vi "Build Name and Value arrays from Variant.vi"(7 "Format String (%#_13g)":string="%.3f", 8 "Error":errorcluster, 11 "Anything":variant) -> (0 "Error Out":errorcluster, 2 "Value Array Out":string[](array[string]), 3 "Name Array Out":string[](array[string]), 5 "Default Section Name Out":string)   [LabVIEW 2020]
uses:
  <vilib>/Utility/Data Type/NI_Data Type.lvlib
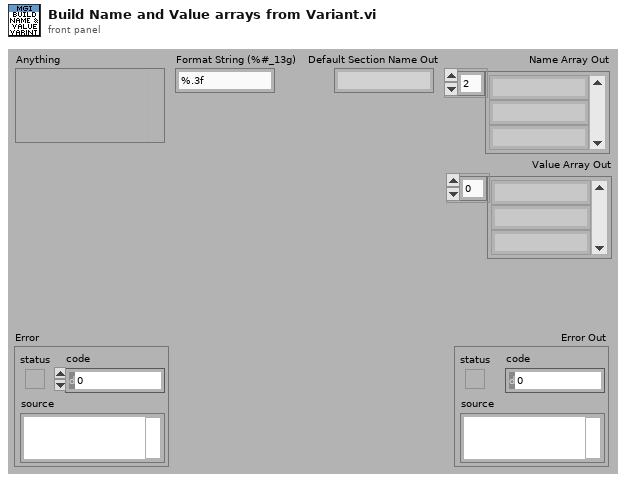
[diagram p1: front panel]
types:
  T1 = typedef "NI_Data Type.lvlib/Data Type.ctl" = enum8{"Invalid Type", "Void", "I8", "I16", "I32", "I64", "U8", "U16", "U32", "U64", "Single Float", "Double Float", "Extended Float", "Single Complex", "Double Complex", "Extended Complex", "Enum U8", "Enum U16", "Enum U32", "Enum U64", "Single Float With Unit", "Double Float With Unit", "Extended Float With Unit", "Single Complex with Unit", "Double Complex with Unit", "Extended Complex with Unit", "Boolean", "String", "Path", "Picture", "Tag", "Array", "Cluster", "Variant", "LV Variant", "Waveform", "Timestamp", "Digital Waveform", "Digital Data", "ExpressData", "Refnum", "External Data", "VI", "Poly VI", "LabVIEW Class Instance", "Fixed Point", "Set Collection", "Map Collection"}
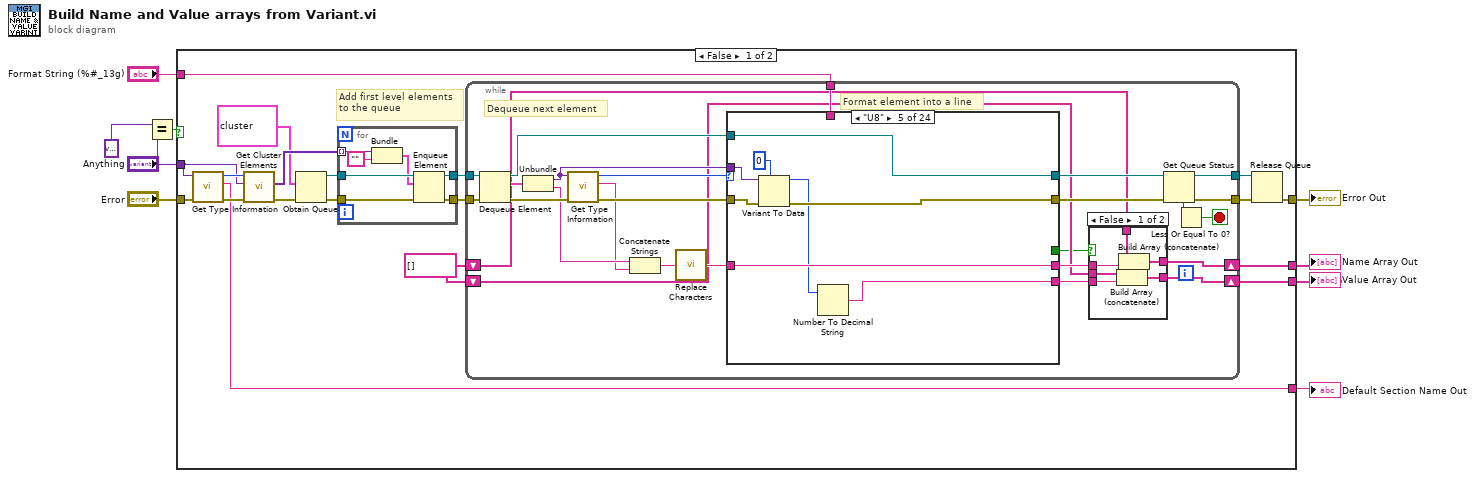
[diagram p0: block diagram]
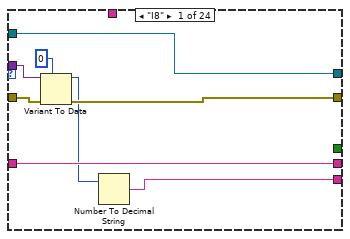
[diagram p3: hidden frame]
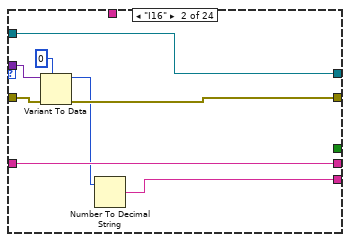
[diagram p4: hidden frame]
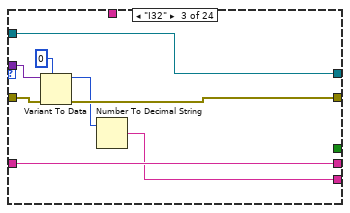
[diagram p5: hidden frame]
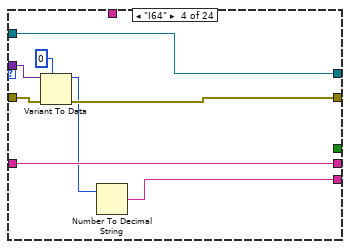
[diagram p6: hidden frame]
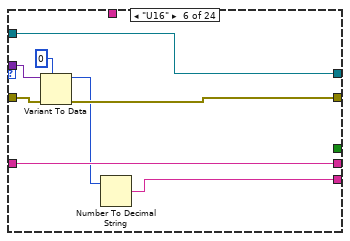
[diagram p7: hidden frame]
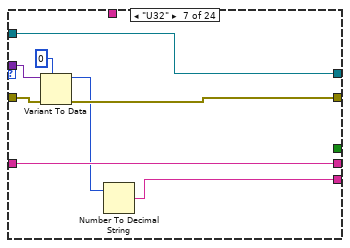
[diagram p8: hidden frame]
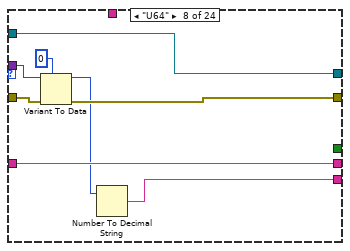
[diagram p9: hidden frame]
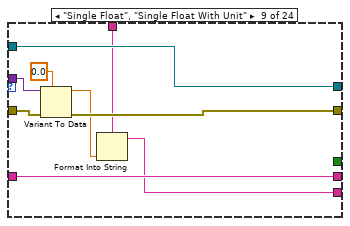
[diagram p10: hidden frame]
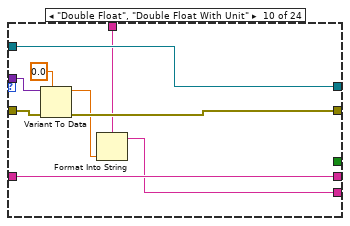
[diagram p11: hidden frame]
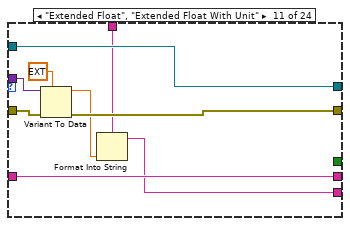
[diagram p12: hidden frame]
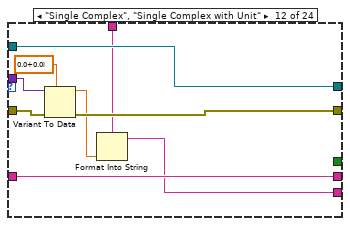
[diagram p13: hidden frame]
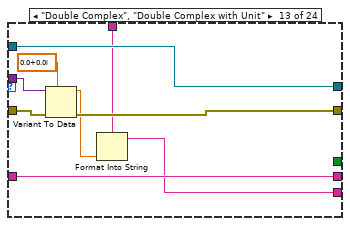
[diagram p14: hidden frame]
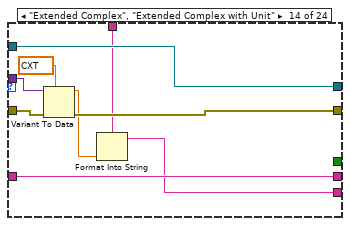
[diagram p15: hidden frame]
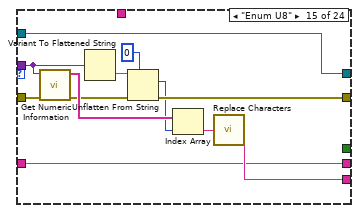
[diagram p16: hidden frame]
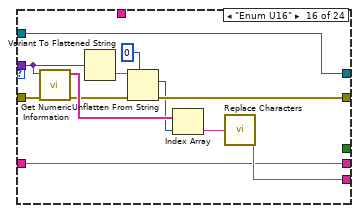
[diagram p17: hidden frame]
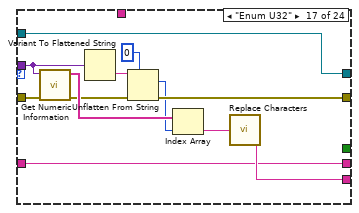
[diagram p18: hidden frame]
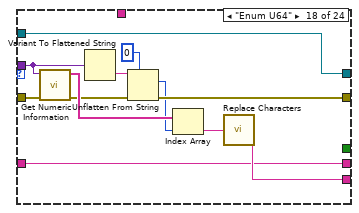
[diagram p19: hidden frame]
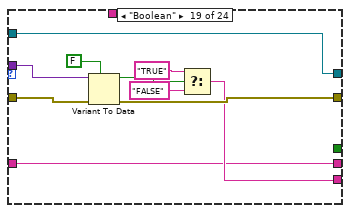
[diagram p20: hidden frame]
diagram:
  n1 = Equal?(x=variant ("Anything"), y="Anything") -> (x = y?=w1:bool)
  n2 = case shown="False" w1 {
    tunnel: [w28 _] -> w9
    tunnel: [w27 _] -> w8
    tunnel: "Error" -> [w26 w301]
    tunnel: "Format String (%#_13g)" -> [w25 _]
    tunnel: [w23 w301] -> w5
    tunnel: [w12 _] -> w4
    tunnel: "Anything" -> [w10 _]
    frame False {
      w11 = string[] []
      # "Add first level elements\nto the queue"
      n3 = call <vilib>:"Get Type Information.vi"("error in (no error)"=w26, "variant"=w10) -> ("error out"=w20:errorcluster, "name"=w12:string, "type"=w24:T1)  [unwired: 5 in, 2 out]
      n4 = call "Get Cluster Elements.vi"("Error In"=w20, "Cluster"=w10, "Type Enum (Cluster)"=w24) -> ("Error Out"=w22:errorcluster, "Cluster Elements"=w21:variant[])  [unwired: 7 in]
      n5 = Obtain Queue(element data type=cluster{"Variant":variant, "Name":string} {"Variant"=variant, "Name"=""}, error in (no error)=w22) -> (queue out=w13:refnum<queue>, error out=w14:errorcluster)  [unwired: 3 in, 1 out]
      n6 = for {
        tunnel: w13 -> [w35]
        tunnel: w14 -> [w34]
        tunnel: [w33] -> w15
        tunnel: [w32] -> w16
        tunnel: w21 -> [w30] mode=indexing
        n7 = Bundle("Variant"=w30, "") -> (w31:cluster{"Variant":variant, string})  [unwired: 1 in]
        n8 = Enqueue Element(queue=w35, element=w31, error in (no error)=w34) -> (queue out=w32:refnum<queue>, error out=w33:errorcluster)  [unwired: 1 in, 1 out]
      }
      n9 = while {
        tunnel: w15 -> [w61]
        tunnel: [w58] -> w17
        tunnel: w16 -> [w59]
        tunnel: [w55] -> w18
        tunnel: w25 -> [w43]
        shift-right: [w40] -> w28
        shift-left: w11 -> [w37]
        shift-right: [w39] -> w27
        shift-left: w11 -> [w38]
        stop <- w56 stop-if-true
        # "Format element into a line"
        # "Dequeue next element"
        n10 = Dequeue Element(queue=w59, error in (no error)=w61) -> (queue out=w52:refnum<queue>, element=w50:cluster{"Variant":variant, "Name":string}, error out=w60:errorcluster)  [unwired: 1 in, 1 out]
        n11 = Unbundle(w50) -> ("Variant"=w49:variant, "Name"=w48:string)
        n12 = call <vilib>:"Get Type Information.vi"("error in (no error)"=w60, "variant"=w49) -> ("error out"=w47:errorcluster, "name"=w46:string, "type"=w54:T1)  [unwired: 5 in, 2 out]
        n13 = Concatenate Strings(w48, w46) -> (w45:string)
        n14 = call "Replace Characters.vi"("String In"=w45) -> ("String Out"=w44:string)  [unwired: 1 in]
        n15 = case shown="\"U8\"" w54 {
          selector: w54 -> [_ _ _ _ _ _ _ _ _ _ _ _ _ _ _ _ _ _ _ _ _ w269 _ _]
          tunnel: [w77 w85 w93 w101 w109 w117 w125 w133 w142 w151 w160 w169 w178 w187 w199 w211 w223 w235 w245 w253 w262 w273 w286 w300] -> w53
          tunnel: w52 -> [w77 w85 w93 w101 w109 w117 w125 w133 w142 w151 w160 w169 w178 w187 w199 w211 w223 w235 w245 w253 w262 w274 w290 w300]
          tunnel: [w73 w81 w89 w97 w105 w113 w121 w129 w138 w147 w156 w165 w174 w183 w193 w205 w217 w229 w244 w252 w261 w275 w287 w299] -> w51
          tunnel: w47 -> [w76 w84 w92 w100 w108 w116 w124 w132 w141 w150 w159 w168 w177 w186 w198 w210 w222 w234 w241 w249 w258 w271 w288 w299]
          tunnel: w44 -> [w72 w80 w88 w96 w104 w112 w120 w128 w135 w144 w153 w162 w171 w180 w188 w200 w212 w224 w236 w246 w254 w265 w283 w291]
          tunnel: w49 -> [w75 w83 w91 w99 w107 w115 w123 w131 w140 w149 w158 w167 w176 w185 w196 w208 w220 w232 w242 w250 w259 w268 w289 w298]
          tunnel: w43 -> [_ _ _ _ _ _ _ _ w136 w145 w154 w163 w172 w181 _ _ _ _ _ _ _ _ w285 _]
          tunnel: [w72 w80 w88 w96 w104 w112 w120 w128 w135 w144 w153 w162 w171 w180 w188 w200 w212 w224 w236 w246 w254 _ w283 w291] -> w42
          tunnel: [w70 w78 w87 w94 w103 w110 w118 w126 w134 w143 w152 w161 w170 w179 w189 w201 w213 w225 w237 w247 w255 _ w284 w292] -> w41
          tunnel: [_ _ _ _ _ _ _ _ _ _ _ _ _ _ _ _ _ _ _ _ _ TRUE _ _] -> w36
          frame "I8" {
            n16 = Variant To Data(error in=w76, type=i8 0, Variant=w75) -> (data=w71:i8, error out=w73:errorcluster)
            n17 = Number To Decimal String(number=w71) -> (decimal integer string=w70:string)  [unwired: 1 in]
          }
          frame "I16" {
            n18 = Variant To Data(error in=w84, type=i16 0, Variant=w83) -> (data=w79:i16, error out=w81:errorcluster)
            n19 = Number To Decimal String(number=w79) -> (decimal integer string=w78:string)  [unwired: 1 in]
          }
          frame "I32" {
            n20 = Variant To Data(error in=w92, type=0, Variant=w91) -> (data=w86:i32, error out=w89:errorcluster)
            n21 = Number To Decimal String(number=w86) -> (decimal integer string=w87:string)  [unwired: 1 in]
          }
          frame "I64" {
            n22 = Variant To Data(error in=w100, type=i64 0, Variant=w99) -> (data=w95:i64, error out=w97:errorcluster)
            n23 = Number To Decimal String(number=w95) -> (decimal integer string=w94:string)  [unwired: 1 in]
          }
          frame "U8" {
            n24 = Variant To Data(error in=w108, type=u8 0, Variant=w107) -> (data=w102:u8, error out=w105:errorcluster)
            n25 = Number To Decimal String(number=w102) -> (decimal integer string=w103:string)  [unwired: 1 in]
          }
          frame "U16" {
            n26 = Variant To Data(error in=w116, type=u16 0, Variant=w115) -> (data=w111:u16, error out=w113:errorcluster)
            n27 = Number To Decimal String(number=w111) -> (decimal integer string=w110:string)  [unwired: 1 in]
          }
          frame "U32" {
            n28 = Variant To Data(error in=w124, type=u32 0, Variant=w123) -> (data=w119:u32, error out=w121:errorcluster)
            n29 = Number To Decimal String(number=w119) -> (decimal integer string=w118:string)  [unwired: 1 in]
          }
          frame "U64" {
            n30 = Variant To Data(error in=w132, type=u64 0, Variant=w131) -> (data=w127:u64, error out=w129:errorcluster)
            n31 = Number To Decimal String(number=w127) -> (decimal integer string=w126:string)  [unwired: 1 in]
          }
          frame "Single Float", "Single Float With Unit" {
            n32 = Variant To Data(error in=w141, type=sgl 0.0, Variant=w140) -> (data=w137:sgl, error out=w138:errorcluster)
            n33 = Format Into String(format string=w136, w137) -> (resulting string=w134:string)  [unwired: 2 in, 1 out]
          }
          frame "Double Float", "Double Float With Unit" {
            n34 = Variant To Data(error in=w150, type=0.0, Variant=w149) -> (data=w146:dbl, error out=w147:errorcluster)
            n35 = Format Into String(format string=w145, w146) -> (resulting string=w143:string)  [unwired: 2 in, 1 out]
          }
          frame "Extended Float", "Extended Float With Unit" {
            n36 = Variant To Data(error in=w159, type=ext 0.0, Variant=w158) -> (data=w155:ext, error out=w156:errorcluster)
            n37 = Format Into String(format string=w154, w155) -> (resulting string=w152:string)  [unwired: 2 in, 1 out]
          }
          frame "Single Complex", "Single Complex with Unit" {
            n38 = Variant To Data(error in=w168, type=csg 0.0+0.0i, Variant=w167) -> (data=w164:csg, error out=w165:errorcluster)
            n39 = Format Into String(format string=w163, w164) -> (resulting string=w161:string)  [unwired: 2 in, 1 out]
          }
          frame "Double Complex", "Double Complex with Unit" {
            n40 = Variant To Data(error in=w177, type=cdb 0.0+0.0i, Variant=w176) -> (data=w173:cdb, error out=w174:errorcluster)
            n41 = Format Into String(format string=w172, w173) -> (resulting string=w170:string)  [unwired: 2 in, 1 out]
          }
          frame "Extended Complex", "Extended Complex with Unit" {
            n42 = Variant To Data(error in=w186, type=cxt 0.0+0.0i, Variant=w185) -> (data=w182:cxt, error out=w183:errorcluster)
            n43 = Format Into String(format string=w181, w182) -> (resulting string=w179:string)  [unwired: 2 in, 1 out]
          }
          frame "Enum U8" {
            n44 = call <vilib>:"Get Numeric Information.vi"("error in (no error)"=w198, "variant"=w196) -> ("error out"=w194:errorcluster, "enum names"=w197:string[])  [unwired: 6 in, 2 out]
            n45 = Variant To Flattened String(Variant=w196) -> (data string=w195:string)  [unwired: 1 out]
            n46 = Unflatten From String(type=u8 0, binary string=w195, error in (no error)=w194) -> (value=w192:u8, error out=w193:errorcluster)  [unwired: 2 in, 1 out]
            n47 = Index Array(array=w197, index=w192) -> (element=w190:string)
            n48 = call "Replace Characters.vi"("String In"=w190) -> ("String Out"=w189:string)  [unwired: 1 in]
          }
          frame "Enum U16" {
            n49 = call <vilib>:"Get Numeric Information.vi"("error in (no error)"=w210, "variant"=w208) -> ("error out"=w206:errorcluster, "enum names"=w209:string[])  [unwired: 6 in, 2 out]
            n50 = Variant To Flattened String(Variant=w208) -> (data string=w207:string)  [unwired: 1 out]
            n51 = Unflatten From String(type=u16 0, binary string=w207, error in (no error)=w206) -> (value=w204:u16, error out=w205:errorcluster)  [unwired: 2 in, 1 out]
            n52 = Index Array(array=w209, index=w204) -> (element=w202:string)
            n53 = call "Replace Characters.vi"("String In"=w202) -> ("String Out"=w201:string)  [unwired: 1 in]
          }
          frame "Enum U32" {
            n54 = call <vilib>:"Get Numeric Information.vi"("error in (no error)"=w222, "variant"=w220) -> ("error out"=w218:errorcluster, "enum names"=w221:string[])  [unwired: 6 in, 2 out]
            n55 = Variant To Flattened String(Variant=w220) -> (data string=w219:string)  [unwired: 1 out]
            n56 = Unflatten From String(type=u32 0, binary string=w219, error in (no error)=w218) -> (value=w216:u32, error out=w217:errorcluster)  [unwired: 2 in, 1 out]
            n57 = Index Array(array=w221, index=w216) -> (element=w214:string)
            n58 = call "Replace Characters.vi"("String In"=w214) -> ("String Out"=w213:string)  [unwired: 1 in]
          }
          frame "Enum U64" {
            n59 = call <vilib>:"Get Numeric Information.vi"("error in (no error)"=w234, "variant"=w232) -> ("error out"=w230:errorcluster, "enum names"=w233:string[])  [unwired: 6 in, 2 out]
            n60 = Variant To Flattened String(Variant=w232) -> (data string=w231:string)  [unwired: 1 out]
            n61 = Unflatten From String(type=u64 0, binary string=w231, error in (no error)=w230) -> (value=w228:u64, error out=w229:errorcluster)  [unwired: 2 in, 1 out]
            n62 = Index Array(array=w233, index=w228) -> (element=w226:string)
            n63 = call "Replace Characters.vi"("String In"=w226) -> ("String Out"=w225:string)  [unwired: 1 in]
          }
          frame "Boolean" {
            n64 = Variant To Data(error in=w241, type=FALSE, Variant=w242) -> (data=w240:bool, error out=w244:errorcluster)
            n65 = Select(t="TRUE", s=w240, f="FALSE") -> (s? t:f=w237:string)
          }
          frame "String" {
            n66 = Variant To Data(error in=w249, type="", Variant=w250) -> (data=w248:string, error out=w252:errorcluster)
            n67 = call "Replace Characters.vi"("String In"=w248) -> ("String Out"=w247:string)  [unwired: 1 in]
          }
          frame "Path" {
            n68 = Variant To Data(error in=w258, type=path "", Variant=w259) -> (data=w257:path, error out=w261:errorcluster)
            n69 = Path To String(path=w257) -> (string=w256:string)
            n70 = call "Replace Characters.vi"("String In"=w256) -> ("String Out"=w255:string)  [unwired: 1 in]
          }
          frame "Cluster" {
            # "Enqueue cluster elements"
            n71 = call "Get Cluster Elements.vi"("Error In"=w271, "Cluster"=w268, "Type Enum (Cluster)"=w269) -> ("Error Out"=w270:errorcluster, "Cluster Elements"=w267:variant[])  [unwired: 7 in]
            n72 = Concatenate Strings(w265, "." ("string")) -> (w264:string)
            n73 = Reverse 1D Array(array=w267) -> (reversed array=w272:variant[])
            n74 = for {
              tunnel: w274 -> [w282]
              tunnel: w270 -> [w281]
              tunnel: [w280] -> w275
              tunnel: [w279] -> w273
              tunnel: w272 -> [w277] mode=indexing
              tunnel: w264 -> [w276]
              n75 = Bundle("Variant"=w277, w276) -> (w278:cluster{"Variant":variant, string})  [unwired: 1 in]
              n76 = Enqueue Element At Opposite End(queue=w282, element=w278, error in (no error)=w281) -> (queue out=w279:refnum<queue>, error out=w280:errorcluster)  [unwired: 1 in, 1 out]
            }
          }
          frame "Array" {
            n77 = call "Process Array Elements.vi"("Format String (%#0.15f)"=w285, "Error In"=w288, "Name In"=w283, "Array Variant"=w289, "Queue In"=w290) -> ("Error Out"=w287:errorcluster, "Data Out"=w284:string, "Queue Out"=w286:refnum<queue>)  [unwired: 4 in]
          }
          frame Default {
            n78 = Variant To Flattened String(Variant=w298) -> (data string=w293:string)  [unwired: 1 out]
            n79 = String To Byte Array(string=w293) -> (unsigned byte array=w297:u8[])
            n80 = Number To Hexadecimal String(1:i16 2 ("width (-)"), 2:w297) -> (0:w296:string[])
            n81 = Concatenate Strings("0x", w296) -> (w292:string)
          }
        }
        n82 = case shown="False" w36 {
          tunnel: w42 -> [w67 _]
          tunnel: w41 -> [w66 _]
          tunnel: [w65 w69] -> w40
          tunnel: [w64 w68] -> w39
          tunnel: w38 -> [w63 w68]
          tunnel: w37 -> [w62 w69]
          frame False {
            n83 = Build Array (concatenate)(w63, w66) -> (w64:string[])
            n84 = Build Array (concatenate)(w62, w67) -> (w65:string[])
          }
          frame True {
          }
        }
        n85 = Get Queue Status(queue=w53, error in (no error)=w51) -> (queue out=w55:refnum<queue>, error out=w58:errorcluster, # elements in queue=w57:i32)  [unwired: 1 in, 5 out]
        n86 = Less Or Equal To 0?(x=w57) -> (x <= 0?=w56:bool)
      }
      n87 = Release Queue(queue=w18, error in (no error)=w17) -> (error out=w23:errorcluster)  [unwired: 1 in, 2 out]
    }
    frame True {
    }
  }
  "Name Array Out" <- w9
  "Value Array Out" <- w8
  "Default Section Name Out" <- w4
  "Error Out" <- w5
